vi "mydaq.vi"() -> ()   [LabVIEW 2019]
uses:
  <vilib>/express/express analysis/Spectral/Block/exnSpectralBlock spectral measurements peak poly.vi
  <vilib>/express/express analysis/Spectral/Block/exnSpectralBlock spectral measurements peak DDT.vi
  <vilib>/express/express analysis/Spectral/XNode/ExpressSpectralMeasurementsBlockNode.xnode
panel:
  in  "Tab Control":T1(tab)
  in  "Boolean":bool
  in  "Master Volume":dbl(slide) scale=0.0..1.0
  in  "Treble":dbl(slide) scale=0.0..1.0
  in  "Master Volume":dbl(slide) scale=0.0..1.0
  in  "Bass":dbl(slide) scale=0.0..1.0
  in  "Mid":dbl(slide) scale=0.0..1.0
  out "Waveform Graph 2":dynamicdata(graph)
  in  "stop":bool
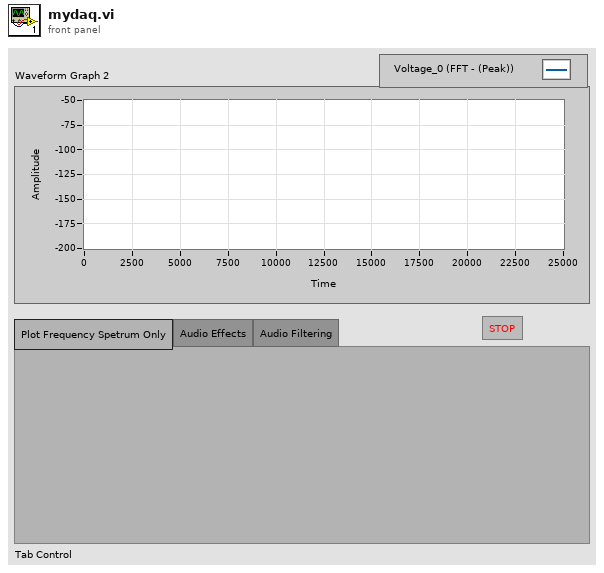
[diagram p1: front panel]
types:
  T1 = enum32{"Plot Frequency Spetrum Only", "Audio Effects", "Audio Filtering"}
  T2 = cluster{"averaging mode":u16, "weighting mode":u16, "number of averages":u32}
  T3 = cluster{"dB On (F)":bool, "unwrap phase (F)":bool, "convert to degree (F)":bool}
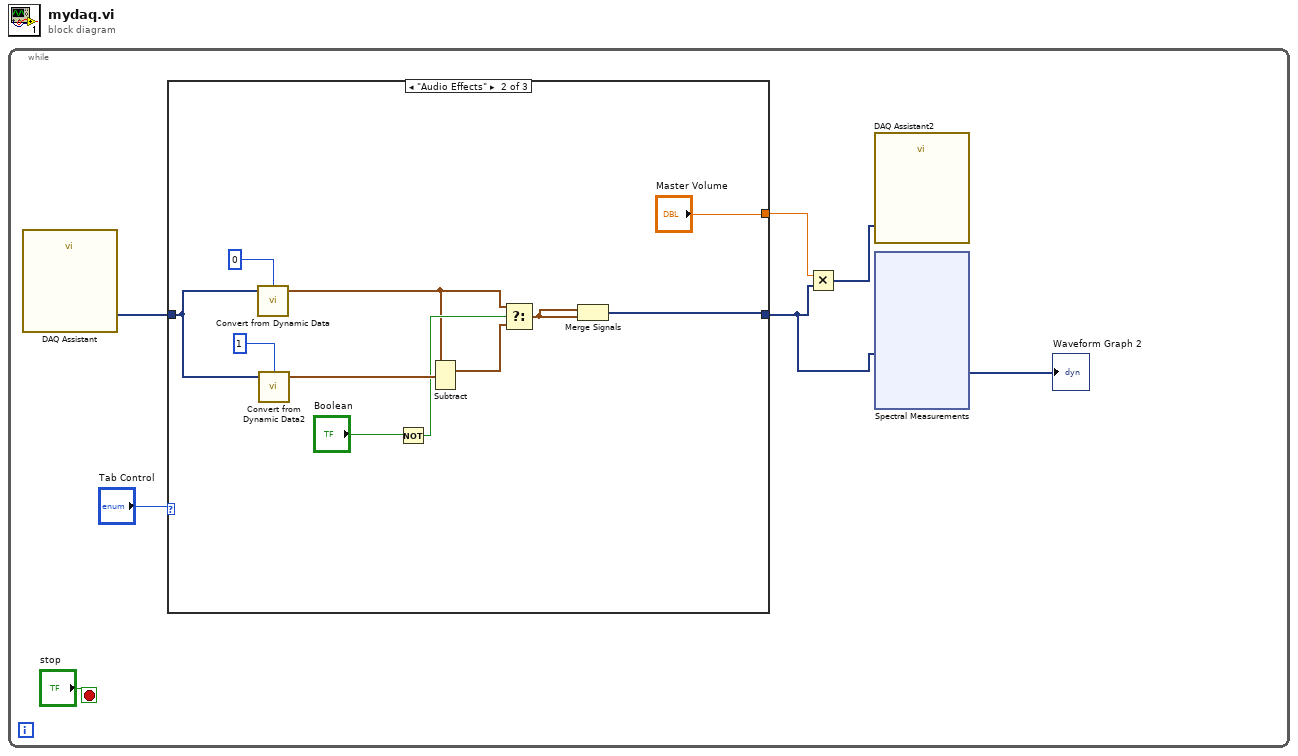
[diagram p0: block diagram]
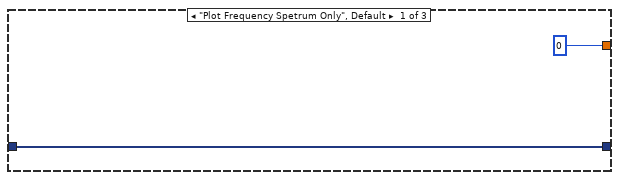
[diagram p2: hidden frame]
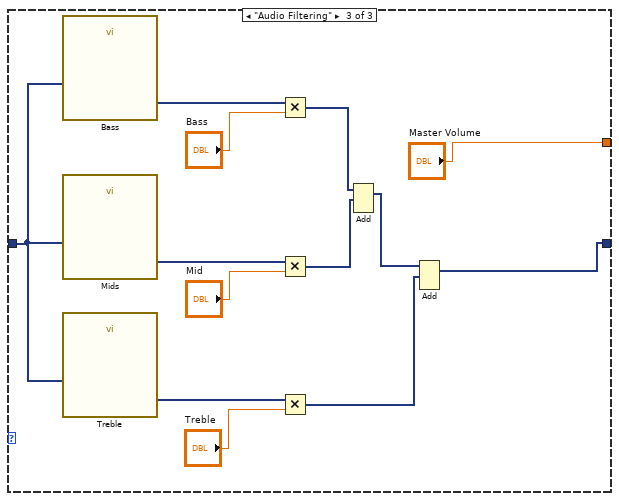
[diagram p3: hidden frame]
diagram:
  n1 = while {
    stop <- "stop" stop-if-true
    n2 = call "DAQ Assistant"() -> ("data"=w5:dynamicdata)  [unwired: 16 in, 3 out]
    n3 = case shown="\"Audio Effects\"" "Tab Control" {
      tunnel: w5 -> [w9 w19 w23]
      tunnel: [w9 w10 w22] -> w3
      tunnel: [0 "Master Volume" "Master Volume"] -> w2
      frame "Plot Frequency Spetrum Only", Default {
      }
      frame "Audio Effects" {
        n4 = call "Convert from Dynamic Data"("Dynamic Data Type"=w19, "Channel"=0) -> ("Waveform"=w12:waveform(dbl))  [unwired: 2 in]
        n5 = call "Convert from Dynamic Data2"("Dynamic Data Type"=w19, "Channel"=1) -> ("Waveform"=w16:waveform(dbl))  [unwired: 2 in]
        n6 = Not(x="Boolean") -> (.not. x?=w13:bool)
        n7 = Subtract(1:w16, 2:w12) -> (0:w14:waveform(dbl))  [unwired: 1 in, 1 out]
        n8 = Select(t=w12, s=w13, f=w14) -> (s? t:f=w11:waveform(dbl))
        n9 = Merge Signals(w11, w11) -> (w10:dynamicdata)
      }
      frame "Audio Filtering" {
        n10 = call "Bass"("Signal"=w23) -> ("Filtered Signal"=w33:dynamicdata)  [unwired: 9 in, 1 out]
        n11 = call "Mids"("Signal"=w23) -> ("Filtered Signal"=w31:dynamicdata)  [unwired: 9 in, 1 out]
        n12 = call "Treble"("Signal"=w23) -> ("Filtered Signal"=w29:dynamicdata)  [unwired: 9 in, 1 out]
        n13 = Multiply(x=w33, y="Bass") -> (x*y=w27:dynamicdata)
        n14 = Multiply(x=w31, y="Mid") -> (x*y=w26:dynamicdata)
        n15 = Multiply(x=w29, y="Treble") -> (x*y=w24:dynamicdata)
        n16 = Add(1:w26, 2:w27) -> (0:w25:dynamicdata)  [unwired: 1 in, 1 out]
        n17 = Add(1:w24, 2:w25) -> (0:w22:dynamicdata)  [unwired: 1 in, 1 out]
      }
    }
    n18 = Multiply(x=w2, y=w3) -> (x*y=w4:dynamicdata)
    n19 = call "DAQ Assistant2"("data"=w4) -> ()  [unwired: 16 in, 3 out]
    n20 = xnode "Spectral Measurements"("Signals"=w3) -> ("FFT - (Peak)"=→"Waveform Graph 2":dynamicdata)  [unwired: 1 in, 2 out]
  }
